vi "230209_Problem.vi"() -> ()   [LabVIEW 2022 SP3]
panel:
  out "Waveform Chart":dbl(graph)
  out "Result":dbl
  in  "stop":bool
  in  "Value 2":dbl(knob) scale=0.0..10.0
  in  "Value 1":dbl(knob) scale=0.0..10.0
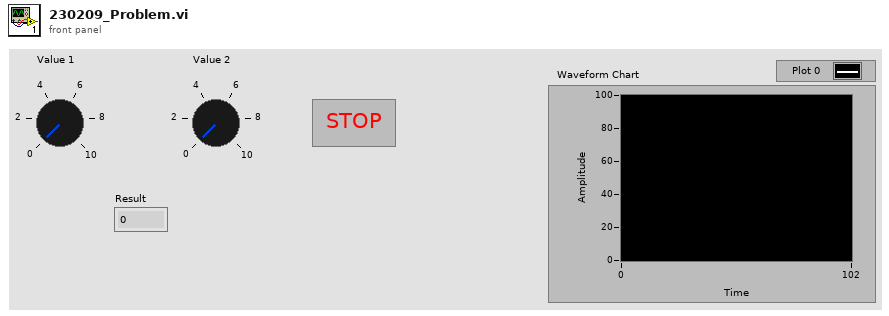
[diagram p1: front panel]
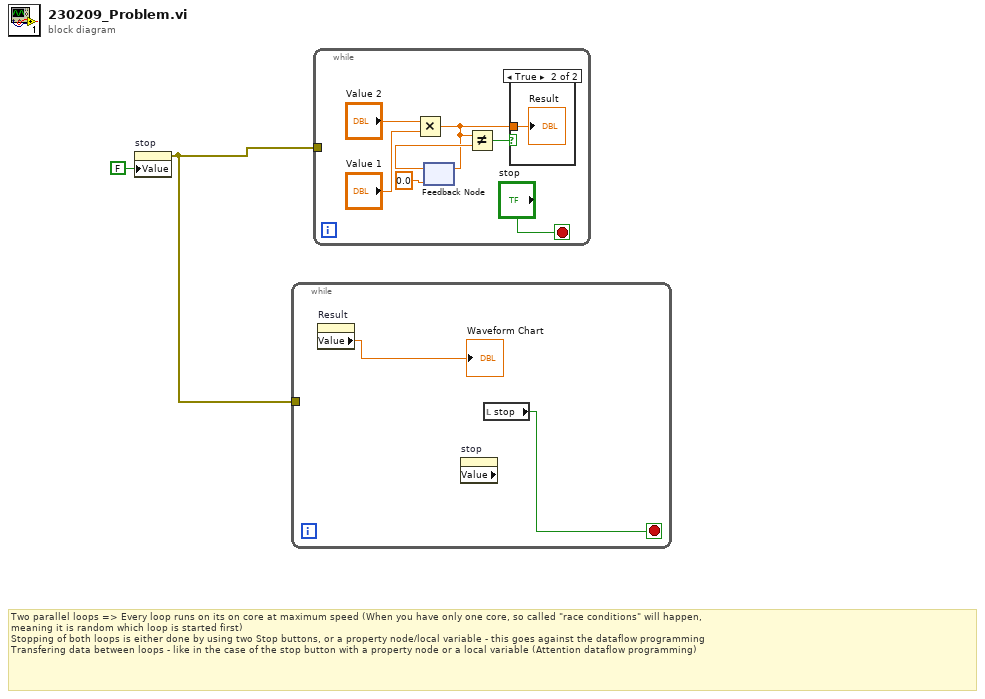
[diagram p0: block diagram]
diagram:
  # "Two parallel loops => Every loop runs on its on core at maximum speed (When you have only one core, so called \"race conditions\" will happen, \nmeaning it is random which loop is started first)\nStopping of both loops is either done by using two Stop buttons, or a property node/local variable - this goes against the dataflow programming\nTransfering data between loops - like in the case of the stop button with a property node or a local variable (Attention dataflow programming)"
  n1 = property on="stop" class="Bool (strict)"("Value"=FALSE ("stop")) -> (error out=w1:errorcluster)  [unwired: 2 in, 1 out]
  n2 = while {
    tunnel: w1 -> [_]
    stop <- w3 stop-if-true
    n3 = property on="Result" class="DigNum (strict)"() -> ("Value"=→"Waveform Chart":dbl)  [unwired: 2 in, 2 out]
    n4 = property on="stop" class="Bool (strict)" props=["Value"]() -> ()  [unwired: 2 in, 3 out]
    n5 = local read "stop"() -> (w3:bool)
  }
  n6 = while {
    tunnel: w1 -> [_]
    stop <- "stop" stop-if-true
    n7 = Multiply(x="Value 2", y="Value 1") -> (x*y=w6:dbl)
    n8 = feedback-in #1(w6) -> ()
    n9 = feedback #1(0.0) -> (w8:dbl)
    n10 = Not Equal?(x=w6, y=w8) -> (x != y?=w7:bool)
    n11 = case shown="True" w7 {
      tunnel: w6 -> [_ w12]
      frame False {
      }
      frame True {
        "Result" <- w12
      }
    }
  }
